vi "calculate number of records.vi"(9 "Resolution":dbl, 10 "Min step":dbl, 11 "Distance":dbl) -> (1 "Resolution records":i32, 2 "Number of records":i32, 3 "Max records":i32)   [LabVIEW 2014]
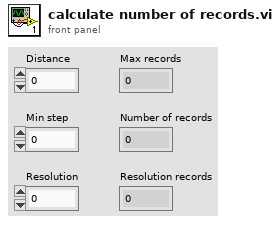
[diagram p1: front panel]
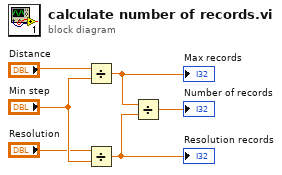
[diagram p0: block diagram]
diagram:
  n1 = Divide(x="Distance", y="Min step") -> (x/y=w6:dbl)
  "Max records" <- w6
  n2 = Divide(x="Resolution", y="Min step") -> (x/y=w4:dbl)
  "Resolution records" <- w4
  n3 = Divide(x=w6, y=w4) -> (x/y=→"Number of records":dbl)
